vi "Get All Endpoint Configurations.vi"(8 "error in (no error)":errorcluster, 11 "Endpoint Configuration Section Ref in":T3 format="%.0x") -> (0 "error out":errorcluster, 2 "All Endpoint Configurations":T1[](array[typedef]), 3 "Endpoint Configuration Section Ref out":T3 format="%.0x")   [LabVIEW 2017, in "SLSC Switch Scripting.lvlib"]
uses:
  SLSC Switch Scripting.lvlib
  <vilib>/NI Veristand/Custom Device API/Custom Device Item Ref.ctl
  Shared/Endpoint Configuration Cluster.ctl
  Shared/Endpoint Configuration Enum.ctl
  <vilib>/NI VeriStand/Custom Device API/Custom Device API.lvlib
  Shared/SLSC Switch Shared.lvlib
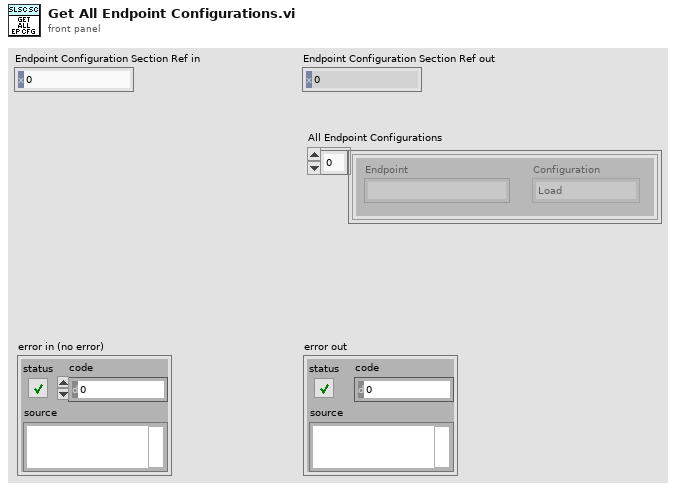
[diagram p1: front panel]
types:
  T1 = typedef "SLSC Switch Shared.lvlib/Endpoint Configuration Cluster.ctl" = cluster{"Endpoint":string, "Configuration":T2}
  T2 = typedef "SLSC Switch Shared.lvlib/Endpoint Configuration Enum.ctl" = enum16{"Load", "Source", "Configuration"}
  T3 = typedef "Custom Device API.lvlib/Custom Device Item Ref.ctl" = u64
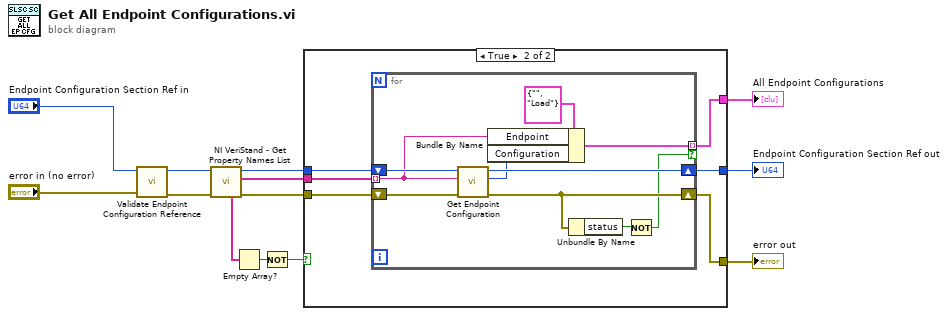
[diagram p0: block diagram]
diagram:
  n1 = call "Validate Endpoint Configuration Reference.vi"("error in (no error)"="error in (no error)", "Endpoint Configuration Section Ref in"="Endpoint Configuration Section Ref in") -> ("error out"=w3:errorcluster, "Endpoint Configuration Section Ref out"=w2:T3)  [unwired: 8 in]
  n2 = call <vilib>:"NI VeriStand - Get Property Names List.vi"("error in (no error)"=w3, "Item Ref in"=w2) -> ("error out"=w10:errorcluster, "Property Names"=w11:string[], "Item Ref out"=w6:T3)  [unwired: 7 in]
  n3 = Empty Array?(array=w11) -> (empty?=w12:bool)
  n4 = Not(x=w12) -> (.not. x?=w4:bool)
  n5 = case shown="True" w4 {
    tunnel: w11 -> [_ w20]
    tunnel: w10 -> [w13 w19]
    tunnel: [_ w18] -> w8
    tunnel: [w13 w17] -> w7
    tunnel: w6 -> [w14 w16]
    tunnel: [w14 w15] -> w5
    frame False {
    }
    frame True {
      n6 = for {
        tunnel: w20 -> [w26] mode=indexing
        shift-right: [w23] -> w17
        shift-left: w19 -> [w27]
        tunnel: [w30] -> w18 mode=indexing if=w21
        shift-right: [w28] -> w15
        shift-left: w16 -> [w29]
        n7 = call "Get Endpoint Configuration.vi"("error in (no error)"=w27, "Endpoint"=w26, "Endpoint Configuration Section Ref in"=w29) -> ("error out"=w23:errorcluster, "Configuration Type"=w25:T2, "Endpoint Configuration Section Ref out"=w28:T3)  [unwired: 6 in]
        n8 = Bundle By Name(cluster=T1 {"Endpoint"="", "Configuration"=enum."Load"} ("Connection"), "Endpoint"=w26, "Configuration"=w25) -> (w30:T1)
        n9 = Unbundle By Name(w23) -> ("status"=w22:bool)
        n10 = Not(x=w22) -> (.not. x?=w21:bool)
      }
    }
  }
  "error out" <- w7
  "Endpoint Configuration Section Ref out" <- w5
  "All Endpoint Configurations" <- w8
